vi "displayConfigurableElements.vi"(11 "ConfigurationThisComponent in":refnum<class "ConfigurationThisComponent.lvclass">) -> (3 "ConfigurationThisComponent out":refnum<class "ConfigurationThisComponent.lvclass">)   [LabVIEW 2013, in "ConfigurationThisComponent.lvclass"]
uses:
  ConfigurationThisComponent.lvclass
  <userlib>/Common/ILC/Configuration/ILC.ctl
  <userlib>/Common/ILC/Configuration/InputChannels.ctl
  <userlib>/Common/ILC/Configuration/ScanRate_Hz_MultichannelOptions.ctl
  <userlib>/Common/SerialProtocols/Configuration/SerialConfig.ctl
  <userlib>/Common/SerialProtocols/Configuration/SerialProtocol.ctl
  <userlib>/Common/SerialProtocols/Configuration/ProtocolParameters.ctl
  <userlib>/Common/SerialProtocols/Configuration/SerialMessageParameters.ctl
  <userlib>/Common/Component/Application/Configuration/Application.ctl
  Configuration/Ambient Temperature Sensor.ctl
  Configuration/Motor Temperature Sensor.ctl
  Configuration/MotorOverheatTemperature.ctl
  Configuration/Distance Gauge.ctl
  Configuration/ChannelsToRead.ctl
  Configuration/Force Sensor.ctl
  Configuration/System Controller.ctl
  Configuration/Stepper Motor.ctl
  <userlib>/Common/ILC/Configuration/ILCConfiguration.lvlib
  <userlib>/Common/SerialProtocols/SerialProtocols.lvlib
  <userlib>/Common/Component/Application/Application.lvlib
panel:
  in  "ctrlRefArrayUsrEvnt":refnum<user-event>
  in  "ConfigTab":T1(tab)
  in  "Application":T2={"Loop Period (ms)"=100} {"Loop Period (ms)" min=1 max=5000}
  in  "ILC":T3={"Input Channels"=enum."Channel 0", "Scan Rate (Hz) "=enum."50", "ADC PGA Gain"=0, "SerialConfig"={"Serial Protocol"=enum."RS485", "Protocol Parameters"={"VISA resource name"="", "Baud Rate"=9600, "Data Bits"=8, "Parity"=enum."None", "Flow Control"=0, "Stop Bits"=10, "Timeout (ms)"=10000}, "Serial Message Parameters"={"Byte Count"=200, "Enable Termination Character"=FALSE, "Termination Char"=200}}} {"SerialConfig"."Serial Message Parameters"."Termination Char" format="%x"; "SerialConfig"."Protocol Parameters"."Stop Bits" items=["1.0"=10, "1.5"=15, "2.0"=20]; "SerialConfig"."Protocol Parameters"."Flow Control" items=["None", "XON/XOFF", "RTS/CTS", "XON/XOFF & RTS/CTS", "DTR/DSR", "XON/XOFF & DTR/DSR"]; "SerialConfig"."Protocol Parameters"."Data Bits" min=5 max=8 step=1; "ADC PGA Gain" max=7}
  in  "Ambient Temperature Sensor":T10={"SerialConfig"={"Serial Protocol"=enum."RS485", "Protocol Parameters"={"VISA resource name"="", "Baud Rate"=9600, "Data Bits"=8, "Parity"=enum."None", "Flow Control"=0, "Stop Bits"=10, "Timeout (ms)"=10000}, "Serial Message Parameters"={"Byte Count"=200, "Enable Termination Character"=FALSE, "Termination Char"=200}}} {"SerialConfig"."Serial Message Parameters"."Termination Char" format="%x"; "SerialConfig"."Protocol Parameters"."Stop Bits" items=["1.0"=10, "1.5"=15, "2.0"=20]; "SerialConfig"."Protocol Parameters"."Flow Control" items=["None", "XON/XOFF", "RTS/CTS", "XON/XOFF & RTS/CTS", "DTR/DSR", "XON/XOFF & DTR/DSR"]; "SerialConfig"."Protocol Parameters"."Data Bits" min=5 max=8 step=1}
  in  "Motor Temperature Sensor":T11={"SerialConfig"={"Serial Protocol"=enum."RS485", "Protocol Parameters"={"VISA resource name"="", "Baud Rate"=9600, "Data Bits"=8, "Parity"=enum."None", "Flow Control"=0, "Stop Bits"=10, "Timeout (ms)"=10000}, "Serial Message Parameters"={"Byte Count"=200, "Enable Termination Character"=FALSE, "Termination Char"=200}}, "Motor Overheat Temperature"=274.15} {"Motor Overheat Temperature" min=274.15 max=573.15 format="%.1f"; "SerialConfig"."Serial Message Parameters"."Termination Char" format="%x"; "SerialConfig"."Protocol Parameters"."Stop Bits" items=["1.0"=10, "1.5"=15, "2.0"=20]; "SerialConfig"."Protocol Parameters"."Flow Control" items=["None", "XON/XOFF", "RTS/CTS", "XON/XOFF & RTS/CTS", "DTR/DSR", "XON/XOFF & DTR/DSR"]; "SerialConfig"."Protocol Parameters"."Data Bits" min=5 max=8 step=1}
  in  "Distance Gauge":T13={"SerialConfig"={"Serial Protocol"=enum."RS485", "Protocol Parameters"={"VISA resource name"="", "Baud Rate"=9600, "Data Bits"=8, "Parity"=enum."None", "Flow Control"=0, "Stop Bits"=10, "Timeout (ms)"=10000}, "Serial Message Parameters"={"Byte Count"=200, "Enable Termination Character"=FALSE, "Termination Char"=200}}, "Channels To Read"=[]} {"SerialConfig"."Serial Message Parameters"."Termination Char" format="%x"; "SerialConfig"."Protocol Parameters"."Stop Bits" items=["1.0"=10, "1.5"=15, "2.0"=20]; "SerialConfig"."Protocol Parameters"."Flow Control" items=["None", "XON/XOFF", "RTS/CTS", "XON/XOFF & RTS/CTS", "DTR/DSR", "XON/XOFF & DTR/DSR"]; "SerialConfig"."Protocol Parameters"."Data Bits" min=5 max=8 step=1}
  in  "Force Sensor":T15={"Force Sensor Conversion"=5000.0} {"Force Sensor Conversion" min=1.0 max=5000000.0 format="%.1f"}
  in  "System Controller":T16={"Per Step Delta Force"=5000.0, "Force Error In Range Limit"=5000.0} {"Force Error In Range Limit" min=10.0 max=5000.0; "Per Step Delta Force" min=1e-05 max=10.0 format="%.3f"}
  in  "Stepper Motor":T17={"Maximum Step Rate"=5000000.0} {"Maximum Step Rate" min=1.0 max=2000.0 format="%.3f"}
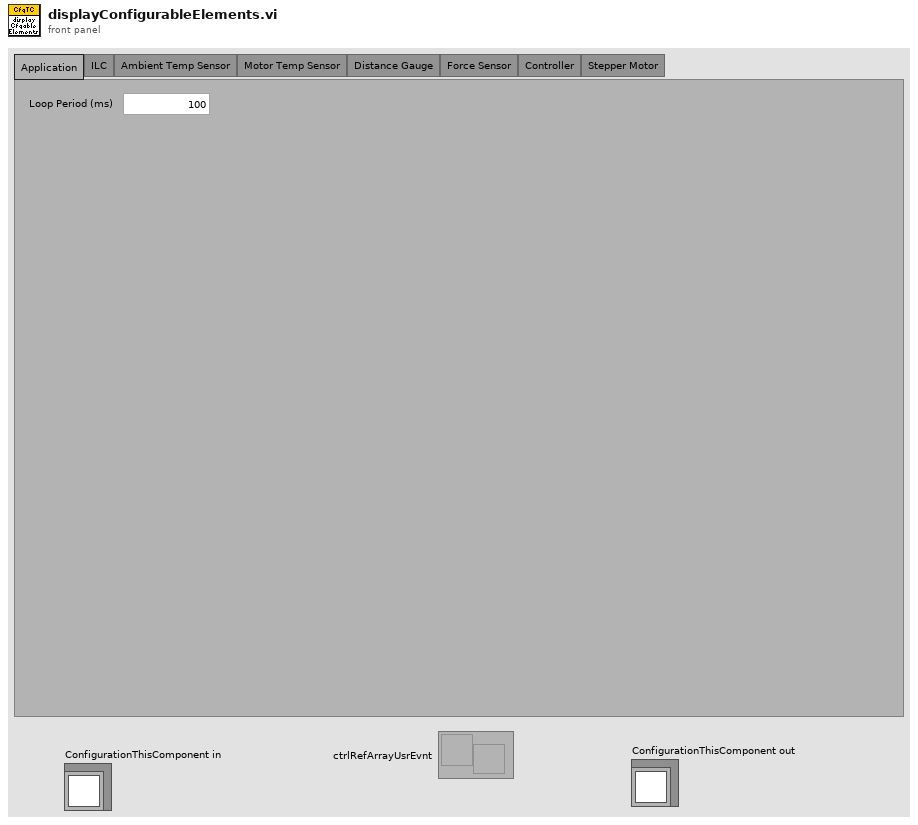
[diagram p1: front panel]
types:
  T1 = enum32{"Application", "ILC", "Ambient Temp Sensor", "Motor Temp Sensor", "Distance Gauge", "Force Sensor", "Controller", "Stepper Motor"}
  T2 = typedef "Application.lvlib/Application.ctl" = cluster{"Loop Period (ms)":u16}
  T3 = typedef "ILCCommon.lvlib/ILCConfiguration.lvlib/ILC.ctl" = cluster{"Input Channels":T4, "Scan Rate (Hz) ":T5, "ADC PGA Gain":u8, "SerialConfig":T6}
  T4 = typedef "ILCCommon.lvlib/ILCConfiguration.lvlib/InputChannels.ctl" = enum16{"Channel 0", "3 Channels", "5 Channels"}
  T5 = typedef "ILCCommon.lvlib/ILCConfiguration.lvlib/ScanRate_Hz_MultichannelOptions.ctl" = enum16{"50", "60", "100", "120", "200", "240", "300", "400", "480", "600", "1200", "2400", "4800"}
  T6 = typedef "SerialProtocols.lvlib/SerialConfig.ctl" = cluster{"Serial Protocol":T7, "Protocol Parameters":T8, "Serial Message Parameters":T9}
  T7 = typedef "SerialProtocols.lvlib/SerialProtocol.ctl" = enum16{"RS232", "RS485", "SerialSimulator"}
  T8 = typedef "SerialProtocols.lvlib/ProtocolParameters.ctl" = cluster{"VISA resource name":refnum<visa-resource-name>, "Baud Rate":u32, "Data Bits":u16, "Parity":enum16{"None", "Odd", "Even", "Mark", "Space"}, "Flow Control":u16, "Stop Bits":u16, "Timeout (ms)":u32}
  T9 = typedef "SerialProtocols.lvlib/SerialMessageParameters.ctl" = cluster{"Byte Count":u32, "Enable Termination Character":bool, "Termination Char":u8}
  T10 = typedef "Ambient Temperature Sensor.ctl" = cluster{"SerialConfig":T6}
  T11 = typedef "Motor Temperature Sensor.ctl" = cluster{"SerialConfig":T6, "Motor Overheat Temperature":T12}
  T12 = typedef "MotorOverheatTemperature.ctl" = dbl[unit]
  T13 = typedef "Distance Gauge.ctl" = cluster{"SerialConfig":T6, "Channels To Read":T14}
  T14 = typedef "ChannelsToRead.ctl" = i32[]
  T15 = typedef "Force Sensor.ctl" = cluster{"Force Sensor Conversion":dbl[unit]}
  T16 = typedef "System Controller.ctl" = cluster{"Per Step Delta Force":dbl[unit], "Force Error In Range Limit":dbl[unit]}
  T17 = typedef "Stepper Motor.ctl" = cluster{"Maximum Step Rate":dbl[unit]}
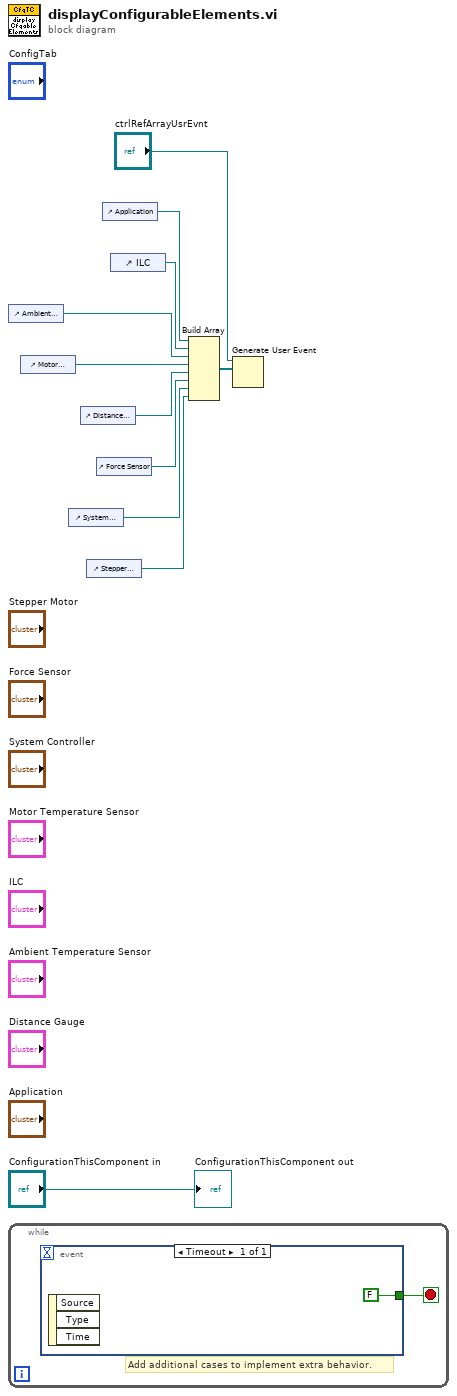
[diagram p0: block diagram]
diagram:
  n1 = control-ref of="Ambient Temperature Sensor"() -> (w6:refnum<vi>)
  n2 = while {
    stop <- w12 stop-if-true
    # "Add additional cases to implement extra behavior."
    n3 = event shown="[0] Timeout" {
      selector: _ -> [_]
      dyn-events: _ -> [_]
      timeout: _ -> [_]
      tunnel: [FALSE] -> w12
      event Timeout {
        n4 = event-data() -> ()  [unwired: 1 in, 3 out]
      }
    }
  }
  n5 = control-ref of="Motor Temperature Sensor"() -> (w5:refnum<vi>)
  n6 = control-ref of="System Controller"() -> (w1:refnum<vi>)
  n7 = control-ref of="Distance Gauge"() -> (w4:refnum<vi>)
  n8 = control-ref of="Stepper Motor"() -> (w2:refnum<vi>)
  n9 = control-ref of="Force Sensor"() -> (w3:refnum<vi>)
  n10 = control-ref of="Application"() -> (w7:refnum<vi>)
  n11 = control-ref of="ILC"() -> (w8:refnum<vi>)
  n12 = Build Array(w7, w8, w6, w5, w4, w3, w1, w2) -> (w11:refnum<vi>[])
  n13 = Generate User Event(user event="ctrlRefArrayUsrEvnt", event data cluster=w11) -> ()  [unwired: 2 in, 2 out]
  "ConfigurationThisComponent out" <- "ConfigurationThisComponent in"
